vi "data to wordarray_EIP.vi"(11 "Data":u8[](array[numeric])) -> (3 "Word array":u16[](array[numeric]))   [LabVIEW 2014]
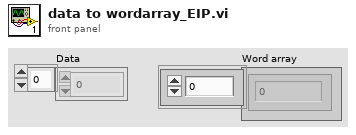
[diagram p1: front panel]
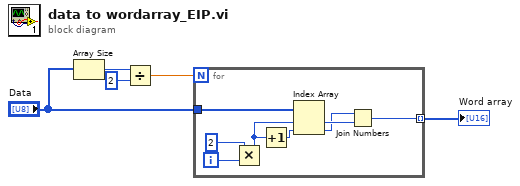
[diagram p0: block diagram]
diagram:
  n1 = Array Size(array="Data") -> (size(s)=w2:i32)
  n2 = Divide(x=w2, y=2) -> (x/y=w4:dbl)
  n3 = for {
    N: w4 -> [_]
    tunnel: "Data" -> [w11]
    tunnel: [w6] -> w5 mode=indexing
    i -> [w13]
    n4 = Multiply(x=2, y=w13) -> (x*y=w10:i32)
    n5 = Increment(x=w10) -> (x+1=w9:i32)
    n6 = Index Array(array=w11, index #1=w10, index #2=w9) -> (element #1=w8:u8, element #2=w7:u8)
    n7 = Join Numbers(hi=w7, lo=w8) -> ((hi.lo)=w6:u16)
  }
  "Word array" <- w5
